vi "Swerve Out of loop.vi"(0 "x":dbl(slide) scale=-1.0..1.0, 1 "Recalc offsets":bool, 2 "Recalc distance":bool=TRUE, 5 "Rot. Point X":dbl, 7 "y":dbl(slide) scale=-1.0..1.0, 9 "Rot. Point Y":dbl, 11 "z":dbl(knob) scale=-1.0..1.0, 12 "Robot Centric":bool=TRUE, 13 "Auto Controls":bool, 14 "Reset Gyro":bool) -> ()   [LabVIEW 2016]
uses:
  <vilib>/Rock Robotics/WPI/ThirdParty/CanMotor/TalonSRX/WPI_CANTalonSRX_APIControlMode.ctl
  <vilib>/Rock Robotics/WPI/ThirdParty/CanMotor/TalonSRX/WPI_CANTalonSRX_APIFeedbackSelect.ctl
  <vilib>/Rock Robotics/Network Tables/NT Read Numeric Array.vi
  Apple Gyro/Apple Pi Gyro Library.lvlib
panel:
  in  "Gyro Select (Overide)":enum16{"IMU", "SPI", "Analog", "Navx", "Pigeon"}(ring)=enum."Pigeon"
  in  "Default Offsets":dbl[](array[numeric])
  in  "negate feedback sensor":bool
  in  "Deadband":dbl=0.04 format="%#_13g"
  in  "Debug?":bool
  in  "Motor":bool[](array[boolean])=[FALSE, FALSE, FALSE, FALSE]
  in  "PIDF":cluster{"P":dbl, "I":dbl, "D":dbl, "F":dbl}={"P"=2.0, "I"=0.0, "D"=0.0, "F"=0.0}
  in  "Robot Width":dbl=26.0
  in  "Robot Length":dbl=22.125
  in  "Override NT?":bool=TRUE
  # "SWERVE DRIVE\nVersion 4.0\nCory Lynch\nChris Garuti\nGavin Popkin\nApple Pi Robotics\nTeam 2067"
  # "FL"
  # "FR"
  # "BL"
  # "BR"
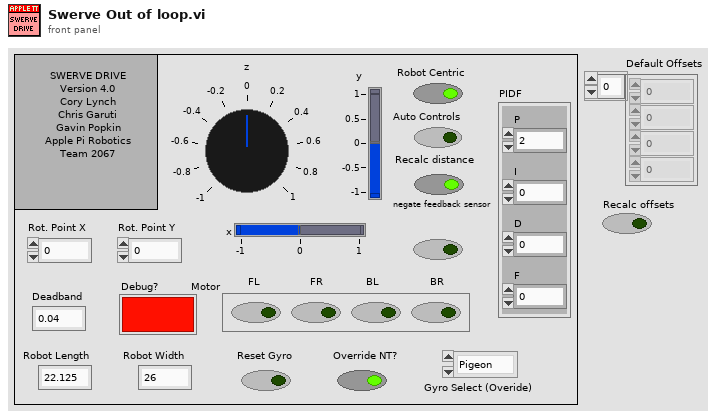
[diagram p1: front panel]
types:
  T1 = typedef "WPI_MotorControlDeviceRef.ctl" = cluster{"DeviceStatus":errorcluster, "Type":T2, "PWM":cluster{"PWM Channel":T3, "DeadBand":T4}, "CAN":cluster{"Device Number":u8, "SetOutput VI Ref":variant, "GetOutput VI Ref":variant, "Enable VI Ref":variant, "Disable VI Ref":variant, "Data":variant}, "Invert":bool}
  T2 = typedef "WPI_MotorControlType.ctl" = enum16{"PWM", "CAN"}
  T3 = typedef "FPGA_DIOPWMChannel.ctl" = enum8{"PWM 0", "PWM 1", "PWM 2", "PWM 3", "PWM 4", "PWM 5", "PWM 6", "PWM 7", "PWM 8", "PWM 9", "PWM MXP 0", "PWM MXP 1", "PWM MXP 2", "PWM MXP 3", "PWM MXP 4", "PWM MXP 5", "PWM MXP 6", "PWM MXP 7", "PWM MXP 8", "PWM MXP 9", "Invalid"}
  T4 = typedef "WPI_PWMDeadband.ctl" = cluster{"Name":string, "maxPositivePwm":i32, "minPositivePwm":i32, "centerPwm":i32, "maxNegativePwm":i32, "minNegativePwm":i32, "angularRange":u16}
  T5 = typedef "WPI_CANTalonSRX_APIFeedbackSelect.ctl" = enum16{"Digital Quadrature Encoder", "Analog Potentiometer", "Analog Encoder", "Count on Quad-A (Rising-Edge)", "Count on Quad-A (Falling-Edge)", "CTR Magnetic Enc (Absolute)", "CTR Magnetic Enc (Relative)", "Pulse Width"}
  T6 = typedef "WPI_CANTalonSRX_GlobalStatus.ctl" = cluster{"Applied Throttle":dbl, "Module Enabled":bool, "CAN Error":errorcluster, "Closed Loop Error":dbl, "Forward Limit Switch Closed":bool, "Reverse Limit Switch Closed":bool, "Sensor Position":dbl, "Sensor Velocity":dbl, "Current":dbl, "Sticky Fault - Over Temp":bool, "Sticky Fault - Under Voltage":bool, "Sticky Fault - Forward Limit":bool, "Sticky Fault - Reverse Limit":bool, "Sticky Fault - Forward Soft Limit":bool, "Sticky Fault - Reverse Soft Limit":bool, "Brake is Enabled":bool, "Encoder Position":dbl, "Encoder Velocity":dbl, "Encoder Index Count":dbl, "Encoder A Pin State":bool, "Encoder B Pin State":bool, "Encoder Index Pin State":bool, "Analog In":dbl, "Analog In Velocity":dbl, "Temperature (C)":dbl, "Battery Voltage":dbl, "Control 5 Is Supported":bool, "Current Profile Slot Select":dbl, "Pos Div 8":bool, "Vel Div 4":bool, "Pulse Width Position":i32, "Pulse Width Velocity":i32, "Pulse Width Rise To Rise (us)":i32, "Pulse Width Rise To Fall (us)":i32, "Mot Prof Active Is Under Run":bool, "Mot Prof Active Has Under Run":bool, "Mot Prof Active Is Last":bool, "Mot Prof Active Velocity Only":bool, "Mot Prof Active Is Valid":bool, "Mot Prof Buffer Is Full":bool, "Mot Prof Active Profile Slot Select":i32, "Mot Prof NextID":i32, "Mot Prof Count":i32, "Mot Prof Active Velocity":dbl, "Mot Prof Active Position":dbl, "Mot Prof Output Enable":i32}
  T7 = typedef "WPI_CANTalonSRX_APIControlMode.ctl" = enum8{"Percent VBus", "Speed", "Position", "Slave", "Unchanged / Invalid", "Voltage Compensation", "Current", "Motion Profile", "Motion Magic"}
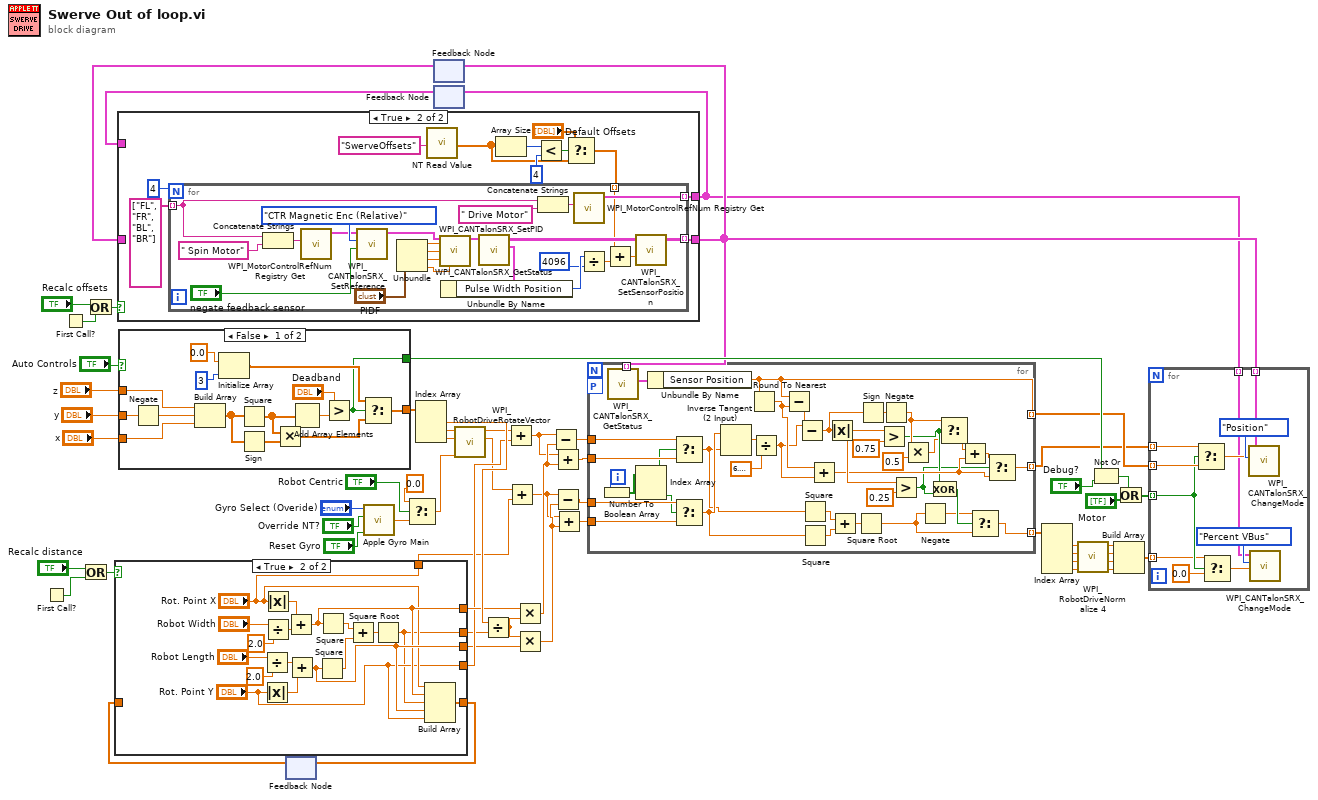
[diagram p0: block diagram]
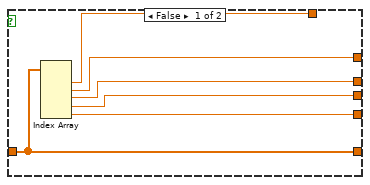
[diagram p3: hidden frame]
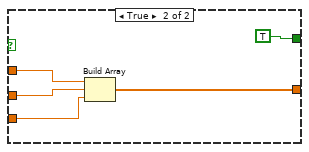
[diagram p4: hidden frame]
diagram:
  n1 = First Call?() -> (First Call?: T/F=w31:bool)
  n2 = First Call?() -> (First Call?: T/F=w1:bool)
  n3 = Or(x="Recalc distance", y=w31) -> (x .or. y?=w29:bool)
  n4 = Or(x="Recalc offsets", y=w1) -> (x .or. y?=w32:bool)
  n5 = case shown="False" "Auto Controls" {
    tunnel: [w69 w80] -> w60
    tunnel: [w65 TRUE] -> w50
    tunnel: "z" -> [w63 w78]
    tunnel: "y" -> [w62 w77]
    tunnel: "x" -> [w61 w76]
    frame False {
      n6 = Negate(x=w62) -> (-x=w64:dbl)
      n7 = Build Array(w63, w64, w61) -> (w73:dbl[])
      n8 = Initialize Array(0.0 ("element"), 3 ("dimension size")) -> (w75:dbl[])
      n9 = Square(x=w73) -> (x^2=w71:dbl[])
      n10 = Sign(1:w73) -> (0:w72:dbl[])
      n11 = Multiply(x=w71, y=w72) -> (x*y=w70:dbl[])
      n12 = Add Array Elements(numeric array=w71) -> (sum=w67:dbl)
      n13 = Greater?(x="Deadband", y=w67) -> (0:w65:bool)
      n14 = Select(t=w75, s=w65, f=w70) -> (s? t:f=w69:dbl[])
    }
    frame True {
      n15 = Build Array(w78, w77, w76) -> (w80:dbl[])
    }
  }
  n16 = feedback #1() -> (w9:dbl[])  [unwired: 1 in]
  n17 = case shown="True" w29 {
    tunnel: [w85 w91] -> w57
    tunnel: [w82 "Rot. Point Y"] -> w56
    tunnel: [w86 "Rot. Point X"] -> w19
    tunnel: [w84 w87] -> w54
    tunnel: [w83 w92] -> w55
    tunnel: [w81 w88] -> w8
    tunnel: w9 -> [w81 _]
    frame False {
      n18 = Index Array(array=w81) -> (element #1=w86:dbl, element #2=w85:dbl, element #3=w84:dbl, element #4=w83:dbl, element #5=w82:dbl)  [unwired: 5 in]
    }
    frame True {
      n19 = Divide(x="Robot Length", y=2.0) -> (x/y=w95:dbl)
      n20 = Absolute Value(x="Rot. Point Y") -> (abs(x)=w94:dbl)
      n21 = Absolute Value(x="Rot. Point X") -> (abs(x)=w93:dbl)
      n22 = Divide(x="Robot Width", y=2.0) -> (x/y=w96:dbl)
      n23 = Add(x=w93, y=w96) -> (x+y=w91:dbl)
      n24 = Add(x=w95, y=w94) -> (x+y=w92:dbl)
      n25 = Square(x=w92) -> (x^2=w98:dbl)
      n26 = Square(x=w91) -> (x^2=w101:dbl)
      n27 = Add(x=w101, y=w98) -> (x+y=w102:dbl)
      n28 = Square Root(x=w102) -> (sqrt(x)=w87:dbl)
      n29 = Build Array("Rot. Point X", w91, w87, w92, "Rot. Point Y") -> (w88:dbl[])
    }
  }
  n30 = feedback-in #1(w8) -> ()
  n31 = call "Apple Gyro Main.vi"("Reset Current"="Reset Gyro", "Override NT?"="Override NT?", "Gyro Select (Overide)"="Gyro Select (Overide)") -> ("Gyro Yaw Out"=w48:dbl)  [unwired: 1 in]
  n32 = Select(t=0.0, s="Robot Centric", f=w48) -> (s? t:f=w44:dbl)
  n33 = Index Array(array=w60) -> (element #1=w59:dbl, element #2=w43:dbl, element #3=w42:dbl)  [unwired: 3 in]
  n34 = feedback #2() -> (w5:T1[])  [unwired: 1 in]
  n35 = feedback #3() -> (w7:T1[])  [unwired: 1 in]
  n36 = case shown="True" w32 {
    tunnel: [w104 w116] -> w6
    tunnel: [w105 w115] -> w4
    tunnel: w7 -> [w105 _]
    tunnel: w5 -> [w104 _]
    frame False {
    }
    frame True {
      n37 = call-poly <vilib>:"NT Read Value.vi"("Name"="SwerveOffsets") -> ("Numeric Array"=w107:dbl[])  [unwired: 9 in, 1 out]
      n38 = Array Size(array=w107) -> (size(s)=w112:i32)
      n39 = Less?(x=w112, y=4) -> (x < y?=w110:bool)
      n40 = Select(t="Default Offsets", s=w110, f=w107) -> (s? t:f=w108:dbl[])
      n41 = for {
        N: 4 -> [_]
        tunnel: string[] ["FL", "FR", "BL", "BR"] -> [w134] mode=indexing
        tunnel: [w131] -> w115 mode=indexing
        tunnel: [w123] -> w116 mode=indexing
        tunnel: w108 -> [w117] mode=indexing
        n42 = Concatenate Strings(w134, " Spin Motor" ("refnum name")) -> (w133:string)
        n43 = call <vilib>:"WPI_MotorControlRefNum Registry Get.vi"("refnum name"=w133) -> ("MotorControlDevRef"=w135:T1)  [unwired: 9 in, 1 out]
        n44 = call <vilib>:"WPI_CANTalonSRX_SetReference.vi"("Reverse Feedback Sensor"="negate feedback sensor", "Feedback Reference"=WPI_CANTalonSRX_APIFeedbackSelect."CTR Magnetic Enc (Relative)", "CAN Talon SRX Ref"=w135) -> ("CAN Talon SRX Ref"=w129:T1)  [unwired: 7 in, 1 out]
        n45 = Unbundle("PIDF") -> ("P"=w136:dbl, "I"=w138:dbl, "D"=w137:dbl, "F"=w127:dbl)
        n46 = call <vilib>:"WPI_CANTalonSRX_SetPID.vi"("CAN Talon SRX Ref"=w129, "P"=w136, "I"=w138, "D"=w137, "F"=w127) -> ("CAN Talon SRX Ref"=w125:T1)  [unwired: 9 in, 1 out]
        n47 = call <vilib>:"WPI_CANTalonSRX_GetStatus.vi"("CAN Talon SRX Ref"=w125) -> ("Talon SRX Status"=w122:T6, "CAN Talon SRX Ref"=w124:T1)  [unwired: 8 in, 1 out]
        n48 = Unbundle By Name(w122) -> ("Pulse Width Position"=w120:i32)
        n49 = Concatenate Strings(w134, " Drive Motor") -> (w132:string)
        n50 = call <vilib>:"WPI_MotorControlRefNum Registry Get.vi"("refnum name"=w132) -> ("MotorControlDevRef"=w131:T1)  [unwired: 9 in, 1 out]
        n51 = Divide(x=w120, y=4096) -> (x/y=w121:dbl)
        n52 = Add(x=w117, y=w121) -> (x+y=w118:dbl)
        n53 = call <vilib>:"WPI_CANTalonSRX_SetSensorPosition.vi"("New Sensor Position"=w118, "CAN Talon SRX Ref"=w124) -> ("CAN Talon SRX Ref"=w123:T1)  [unwired: 8 in, 1 out]
      }
    }
  }
  n54 = feedback-in #2(w6) -> ()
  n55 = feedback-in #3(w4) -> ()
  n56 = call <vilib>:"WPI_RobotDriveRotateVector.vi"("Angle"=w44, "X"=w42, "Y"=w43) -> ("X'"=w40:dbl, "Y'"=w41:dbl)  [unwired: 7 out]
  n57 = Divide(x=w59, y=w54) -> (x/y=w58:dbl)
  n58 = Add(x=w41, y=w56) -> (x+y=w20:dbl)
  n59 = Add(x=w40, y=w19) -> (x+y=w21:dbl)
  n60 = Multiply(x=w57, y=w58) -> (x*y=w23:dbl)
  n61 = Multiply(x=w58, y=w55) -> (x*y=w22:dbl)
  n62 = Subtract(x=w20, y=w23) -> (x-y=w27:dbl)
  n63 = Add(x=w20, y=w23) -> (x+y=w26:dbl)
  n64 = Subtract(x=w21, y=w22) -> (x-y=w25:dbl)
  n65 = Add(x=w21, y=w22) -> (x+y=w24:dbl)
  n66 = for {
    tunnel: [w175] -> w18 mode=indexing
    tunnel: [w152] -> w13 mode=indexing
    tunnel: w6 -> [w172] mode=indexing
    tunnel: [w159] -> w28 mode=indexing
    workers-P: _ -> [_]
    tunnel: w27 -> [w166]
    tunnel: w26 -> [w167]
    tunnel: w25 -> [w169]
    tunnel: w24 -> [w168]
    i -> [w171]
    n67 = Number To Boolean Array(number=w171) -> (Boolean array=w170:bool[])
    n68 = call <vilib>:"WPI_CANTalonSRX_GetStatus.vi"("CAN Talon SRX Ref"=w172) -> ("Talon SRX Status"=w144:T6)  [unwired: 8 in, 2 out]
    n69 = Index Array(array=w170) -> (element #1=w142:bool, element #2=w141:bool)  [unwired: 2 in]
    n70 = Unbundle By Name(w144) -> ("Sensor Position"=w159:dbl)
    n71 = Select(t=w166, s=w142, f=w167) -> (s? t:f=w164:dbl)
    n72 = Select(t=w169, s=w141, f=w168) -> (s? t:f=w165:dbl)
    n73 = Inverse Tangent (2 Input)(1:w164, 2:w165) -> (0:w173:dbl)
    n74 = Round To Nearest(number=w159) -> (nearest integer value=w157:dbl)
    n75 = Divide(x=w173, y=6.283185307179586) -> (x/y=w156:dbl)
    n76 = Subtract(x=w159, y=w157) -> (x-y=w163:dbl)
    n77 = Subtract(x=w156, y=w163) -> (x-y=w158:dbl)
    n78 = Square(x=w164) -> (x^2=w178:dbl)
    n79 = Square(x=w165) -> (x^2=w179:dbl)
    n80 = Add(x=w157, y=w156) -> (x+y=w151:dbl)
    n81 = Absolute Value(x=w158) -> (abs(x)=w161:dbl)
    n82 = Add(x=w178, y=w179) -> (x+y=w177:dbl)
    n83 = Square Root(x=w177) -> (sqrt(x)=w176:dbl)
    n84 = Sign(1:w158) -> (0:w154:dbl)
    n85 = Greater?(x=w161, y=0.75) -> (0:w149:bool)
    n86 = Negate(x=w154) -> (-x=w150:dbl)
    n87 = Greater?(x=w161, y=0.25) -> (0:w143:bool)
    n88 = Multiply(x=w150, y=0.5) -> (x*y=w147:dbl)
    n89 = Negate(x=w176) -> (-x=w145:dbl)
    n90 = Exclusive Or(1:w143, 2:w149) -> (0:w148:bool)
    n91 = Select(t=w150, s=w149, f=w147) -> (s? t:f=w153:dbl)
    n92 = Add(x=w153, y=w151) -> (x+y=w146:dbl)
    n93 = Select(t=w145, s=w148, f=w176) -> (s? t:f=w175:dbl)
    n94 = Select(t=w146, s=w143, f=w151) -> (s? t:f=w152:dbl)
  }
  n95 = Index Array(array=w18) -> (element #1=w17:dbl, element #2=w16:dbl, element #3=w15:dbl, element #4=w14:dbl)  [unwired: 4 in]
  n96 = call <vilib>:"WPI_RobotDriveNormalize 4.vi"("D"=w14, "C"=w15, "B"=w16, "A"=w17) -> ("D'"=w36:dbl, "C'"=w35:dbl, "B'"=w34:dbl, "A'"=w37:dbl)
  n97 = Not Or(1:"Debug?", 2:w50) -> (0:w49:bool)
  n98 = Build Array(w37, w34, w35, w36) -> (w33:dbl[])
  n99 = Or(x=w49, y="Motor") -> (x .or. y?=w53:bool[])
  n100 = for {
    tunnel: w13 -> [w183] mode=indexing
    tunnel: w6 -> [w190] mode=indexing
    tunnel: w53 -> [w182] mode=indexing
    tunnel: w28 -> [w186] mode=indexing
    tunnel: w33 -> [w181] mode=indexing
    tunnel: w4 -> [w180] mode=indexing
    n101 = Select(t=w183, s=w182, f=w186) -> (s? t:f=w185:dbl)
    n102 = Select(t=w181, s=w182, f=0.0) -> (s? t:f=w189:dbl)
    n103 = call <vilib>:"WPI_CANTalonSRX_ChangeMode.vi"("Output"=w185, "Control Mode"=WPI_CANTalonSRX_APIControlMode."Position", "CAN Talon SRX Ref"=w190) -> ()  [unwired: 7 in, 2 out]
    n104 = call <vilib>:"WPI_CANTalonSRX_ChangeMode.vi"("Output"=w189, "Control Mode"=WPI_CANTalonSRX_APIControlMode."Percent VBus", "CAN Talon SRX Ref"=w180) -> ()  [unwired: 7 in, 2 out]
  }
